vi "DeInit.vi"(8 "error in (no error)":errorcluster, 11 "Inovance_Camera in":refnum<class "Inovance_Camera.lvclass">) -> (0 "error out":errorcluster, 3 "Inovance_Camera out":refnum<class "Inovance_Camera.lvclass">)   [LabVIEW 2023, in "Inovance_Camera.lvlib" / "Inovance_Camera.lvclass"]
uses:
  Inovance_Camera.lvclass
  C:/Program Files/National Instruments/LabVIEW 2023/vi.lib/ActorFramework/Actor/Actor.lvclass
  <vilib>/userDefined/High Color/IMAQdx.ctl
  <vilib>/ActorFramework/Actor/Actor.lvclass/Actor.ctl
  Inovance_Camera.lvclass/Inovance_Camera.ctl
  Interfaces/InitDeinitInterface/InitDeinitComm Messages/DeInit Done Msg/DeInit Done Msg.lvclass/DeInit Done Msg.ctl
  <vilib>/ActorFramework/Message Enqueuer/Message Enqueuer.lvclass/Message Enqueuer.ctl
  <vilib>/ActorFramework/Message Enqueuer/Enqueue.vi
  Interfaces/InitDeinitInterface/InitDeinitComm Messages/DeInit Done Msg/DeInit Done Msg.lvclass
  C:/Program Files/National Instruments/LabVIEW 2023/vi.lib/ActorFramework/Message/Message.lvclass
  <vilib>/ActorFramework/Message Priority Queue/Priority Enqueue.vi
  <vilib>/ActorFramework/Actor/Actor.lvclass
  <vilib>/vision/driver/NI_Vision_Acquisition_Software.lvlib
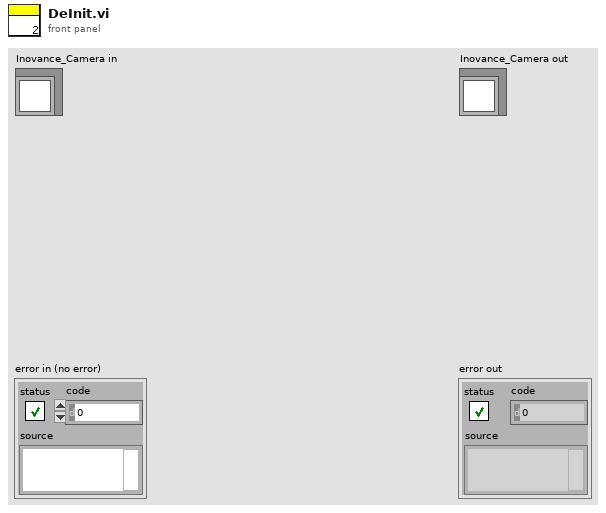
[diagram p1: front panel]
types:
  T1 = typedef "IMAQdx.ctl" = refnum<k21>
  T2 = typedef "typedefs.lvlib/InstrumentData.ctl" = cluster{"Instr Error":errorcluster, "Address":cluster{"address type":enum16{"VISA", "Index"}, "Address":string, "instrument type":T3}, "CurrentState":cluster{"Initialized":bool, "Connected":bool, "Running":bool, "Error":bool}}
  T3 = typedef "typedefs.lvlib/instrumentType.ctl" = enum16{"Spectrometer", "Camera", "Stepper", "Piezo", "SLM"}
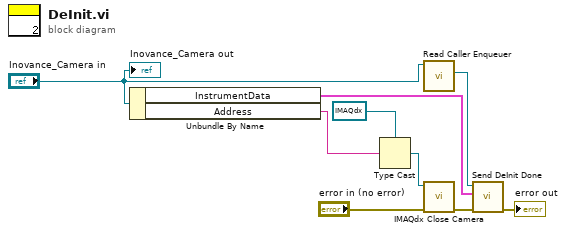
[diagram p0: block diagram]
diagram:
  n1 = Unbundle By Name("Inovance_Camera in") -> ("InstrumentData"=w8:T2, "Address"=w2:string)
  n2 = Type Cast(type=T1 refnum ("Session In"), x=w2) -> (*(type *) &x=w3:T1)
  n3 = call <vilib>:"Read Caller Enqueuer.vi"("Actor"="Inovance_Camera in") -> ("Caller Enqueuer"=w9:refnum<class "Message Enqueuer.lvclass">)  [unwired: 10 in]
  n4 = call <vilib>:"IMAQdx Close Camera.vi"("error in"="error in (no error)", "Session In"=w3) -> ("error out"=w5:errorcluster)  [unwired: 9 in]
  n5 = call "Send DeInit Done.vi"("error in (no error)"=w5, "InstrumentData"=w8, "Message Enqueuer"=w9) -> ("error out"=→"error out":errorcluster)  [unwired: 7 in, 1 out]
  "Inovance_Camera out" <- "Inovance_Camera in"
